vi "SolutionCalculator (SubVI) (2).vi"(4 "Iterative?":bool, 5 "Max Iteration Count":dbl=2.0, 6 "Base Run (matrix)":T1, 7 "Response Coefficients":cdb[][](array[numeric])) -> (0 "Max Residual":dbl, 1 "Correction Phase (radians)":T2, 2 "RMS Residual":dbl format="%0.2f", 3 "Correction Mag":T2)   [LabVIEW 2012]
uses:
  <vilib>/Analysis/Matrix/Datatypes/ComplexMatrix.ctl
  <vilib>/Analysis/Matrix/Datatypes/RealMatrix.ctl
  <vilib>/Analysis/baseanly.llb/Complex A x B.vi
  <vilib>/Analysis/baseanly.llb/Complex Inverse Matrix.vi
  <vilib>/Analysis/Matrix/Numeric/Add/Add - CM,CM.vi
  <vilib>/Analysis/Matrix/Numeric/Conversions/Matrix To Array - CM.vi
  <vilib>/Analysis/5stat.llb/RMS (DBL).vi
  <vilib>/Analysis/Matrix/Numeric/Complex/Complex To Polar - CM.vi
  <vilib>/Analysis/Matrix/Numeric/Absolute Value/Absolute Value - CM.vi
  <vilib>/Analysis/NI_AALBase.lvlib
  <vilib>/Analysis/Matrix/NI_Matrix.lvlib
  <vilib>/Analysis/NI_AALPro.lvlib
panel:
  out "A x B":T1
  out "Epsilon/R":T2
  out "Epsilon":T1
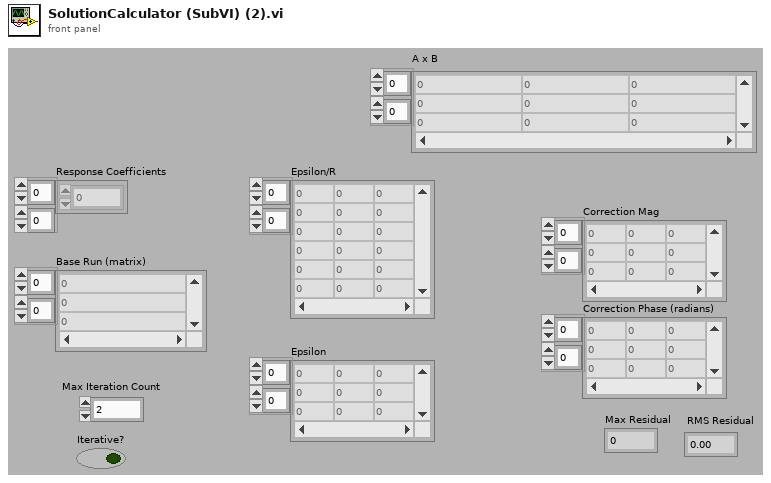
[diagram p1: front panel]
types:
  T1 = typedef "NI_Matrix.lvlib/ComplexMatrix.ctl" = cdb[][]
  T2 = typedef "NI_Matrix.lvlib/RealMatrix.ctl" = dbl[][]
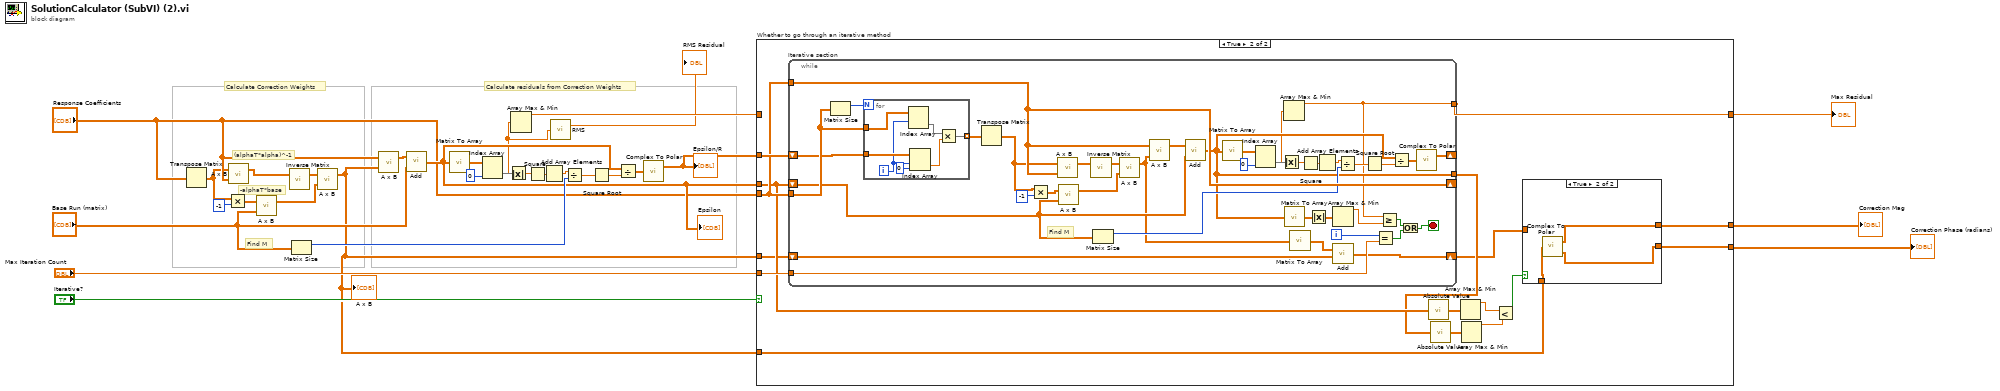
[diagram p0: block diagram]
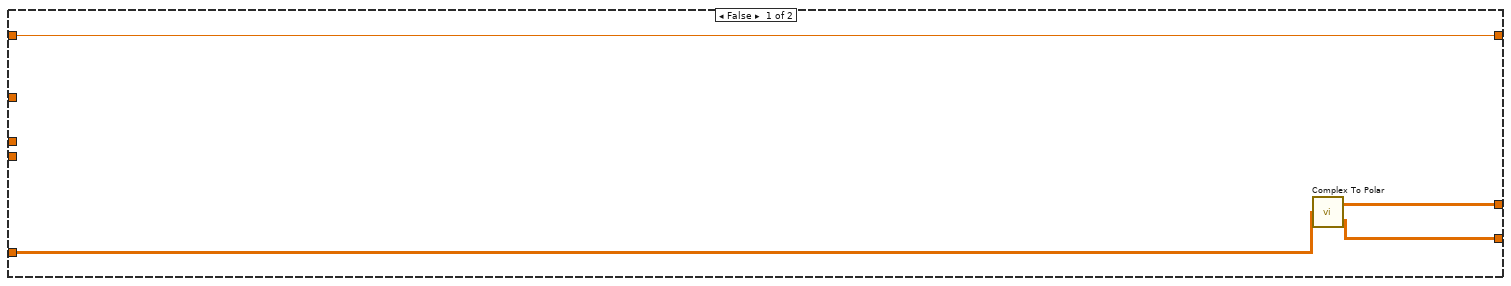
[diagram p2: hidden frame]
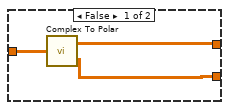
[diagram p3: hidden frame]
diagram:
  # "Calculate residuals from Correction Weights"
  # "Calculate Correction Weights"
  # "-alphaT*base"
  # "(alphaT*alpha)^-1"
  # "Find M"
  n1 = Transpose Matrix(1:"Response Coefficients") -> (0:w6:cdb[][])
  n2 = Multiply ("Multiply.vi")(x=w6, y=-1) -> (x*y=w5:cdb[][])
  n3 = call-poly <vilib>:"A x B.vi"("B"="Response Coefficients", "A"=w6) -> ("A x B"=w4:T1)  [unwired: 1 out]
  n4 = call-poly <vilib>:"A x B.vi"("B"="Base Run (matrix)", "A"=w5) -> ("A x B"=w18:T1)  [unwired: 1 out]
  n5 = call-poly <vilib>:"Inverse Matrix.vi"("Input Matrix"=w4) -> ("Inverse Matrix"=w17:T1)  [unwired: 1 in, 1 out]
  n6 = Matrix Size(0:"Base Run (matrix)") -> (1:w29:i32)  [unwired: 1 out]
  n7 = call-poly <vilib>:"A x B.vi"("B"=w18, "A"=w17) -> ("A x B"=w3:T1)  [unwired: 1 out]
  "A x B" <- w3
  n8 = call-poly <vilib>:"A x B.vi"("B"=w3, "A"="Response Coefficients") -> ("A x B"=w19:T1)  [unwired: 1 out]
  n9 = call-poly <vilib>:"Add.vi"("Complex Matrix B"="Base Run (matrix)", "Complex Matrix A"=w19) -> ("A + B"=w14:T1)
  "Epsilon" <- w14
  n10 = call-poly <vilib>:"Matrix To Array.vi"("Complex Matrix"=w14) -> ("Complex 2D Array"=w20:cdb[][])
  n11 = Index Array(array=w20, index (col)=0 ("disabled index (col)")) -> (element=w27:cdb[])  [unwired: 1 in]
  n12 = Absolute Value(x=w27) -> (abs(x)=w2:dbl[])
  n13 = Array Max & Min(array=w2) -> (max value=w11:dbl)  [unwired: 3 out]
  n14 = Square(x=w2) -> (x^2=w22:dbl[])
  n15 = Add Array Elements(numeric array=w22) -> (sum=w23:dbl)
  n16 = call-poly <vilib>:"RMS.vi"("X"=w2) -> ("rms value"=→"RMS Residual":dbl)  [unwired: 1 out]
  n17 = Divide(x=w23, y=w29) -> (x/y=w24:dbl)
  n18 = Square Root(x=w24) -> (sqrt(x)=w25:dbl)
  n19 = Divide(x=w14, y=w25) -> (x/y=w26:T1)
  n20 = call-poly <vilib>:"Complex To Polar.vi"("Complex Matrix r*e^iQ"=w26) -> ("Modulus r"=w15:T2)  [unwired: 1 out]
  "Epsilon/R" <- w15
  n21 = case "Whether to go through an iterative method" shown="True" "Iterative?" {
    tunnel: "Max Iteration Count" -> [_ w49]
    tunnel: w15 -> [_ w48]
    tunnel: w14 -> [_ w40]
    tunnel: "Response Coefficients" -> [_ w47]
    tunnel: w11 -> [w33 _]
    tunnel: [w33 w46] -> w10
    tunnel: w3 -> [w32 w35]
    tunnel: [w31 w37] -> w9
    tunnel: [w30 w36] -> w8
    tunnel: w3 -> [_ w34]
    frame False {
      n22 = call-poly <vilib>:"Complex To Polar.vi"("Complex Matrix r*e^iQ"=w32) -> ("Modulus r"=w31:T2, "Argument Q"=w30:T2)
    }
    frame True {
      n23 = while "Iterative section" {
        tunnel: w47 -> [w91]
        shift-right: [w65] -> _
        shift-left: w48 -> [w90]
        shift-right: [w66] -> _
        shift-left: w40 -> [w67]
        shift-right: [w80] -> w38
        shift-left: w35 -> [w79]
        tunnel: w49 -> [w81]
        tunnel: w47 -> [w66]
        tunnel: [w61] -> w46
        tunnel: [w63] -> w39
        i -> [w83]
        stop <- w82 stop-if-true
        # "Find M"
        n24 = Matrix Size(0:w91) -> (1:w93:i32)  [unwired: 1 out]
        n25 = for {
          N: w93 -> [_]
          tunnel: w91 -> [w97]
          tunnel: w90 -> [w100]
          tunnel: [w98] -> w92 mode=indexing
          i -> [w94]
          n26 = Index Array(array=w97, index (row)=w94) -> (element=w96:cdb[])  [unwired: 1 in]
          n27 = Index Array(array=w100, index (row)=w94, index (col)=0 ("disabled index (col)")) -> (element=w99:dbl)
          n28 = Multiply(x=w96, y=w99) -> (x*y=w98:cdb[])
        }
        n29 = Transpose Matrix(1:w92) -> (0:w57:cdb[][])
        n30 = Multiply ("Multiply.vi")(x=w57, y=-1) -> (x*y=w59:cdb[][])
        n31 = call-poly <vilib>:"A x B.vi"("B"=w66, "A"=w57) -> ("A x B"=w58:T1)  [unwired: 1 out]
        n32 = call-poly <vilib>:"A x B.vi"("B"=w67, "A"=w59) -> ("A x B"=w77:T1)  [unwired: 1 out]
        n33 = call-poly <vilib>:"Inverse Matrix.vi"("Input Matrix"=w58) -> ("Inverse Matrix"=w78:T1)  [unwired: 1 in, 1 out]
        n34 = Matrix Size(0:w67) -> (1:w64:i32)  [unwired: 1 out]
        n35 = call-poly <vilib>:"A x B.vi"("B"=w77, "A"=w78) -> ("A x B"=w62:T1)  [unwired: 1 out]
        n36 = call-poly <vilib>:"A x B.vi"("B"=w62, "A"=w66) -> ("A x B"=w76:T1)  [unwired: 1 out]
        n37 = call-poly <vilib>:"Add.vi"("Complex Matrix B"=w67, "Complex Matrix A"=w76) -> ("A + B"=w63:T1)
        n38 = call-poly <vilib>:"Matrix To Array.vi"("Complex Matrix"=w63) -> ("Complex 2D Array"=w75:cdb[][])
        n39 = Index Array(array=w75, index (col)=0 ("disabled index (col)")) -> (element=w68:cdb[])  [unwired: 1 in]
        n40 = Absolute Value(x=w68) -> (abs(x)=w56:dbl[])
        n41 = Array Max & Min(array=w56) -> (max value=w61:dbl)  [unwired: 3 out]
        n42 = call-poly <vilib>:"Matrix To Array.vi"("Complex Matrix"=w63) -> ("Complex 2D Array"=w85:cdb[][])
        n43 = call-poly <vilib>:"Matrix To Array.vi"("Complex Matrix"=w62) -> ("Complex 2D Array"=w84:cdb[][])
        n44 = Square(x=w56) -> (x^2=w73:dbl[])
        n45 = Absolute Value(x=w85) -> (abs(x)=w86:dbl[][])
        n46 = Add Array Elements(numeric array=w73) -> (sum=w72:dbl)
        n47 = Array Max & Min(array=w86) -> (max value=w89:dbl)  [unwired: 3 out]
        n48 = call-poly <vilib>:"Add.vi"("Complex Matrix B"=w79, "Complex Matrix A"=w84) -> ("A + B"=w80:T1)
        n49 = Divide(x=w72, y=w64) -> (x/y=w71:dbl)
        n50 = Square Root(x=w71) -> (sqrt(x)=w70:dbl)
        n51 = Equal?(x=w83, y=w81) -> (x = y?=w88:bool)
        n52 = Greater Or Equal?(x=w61, y=w89) -> (x >= y?=w87:bool)
        n53 = Divide(x=w63, y=w70) -> (x/y=w69:T1)
        n54 = Or(x=w87, y=w88) -> (x .or. y?=w82:bool)
        n55 = call-poly <vilib>:"Complex To Polar.vi"("Complex Matrix r*e^iQ"=w69) -> ("Modulus r"=w65:T2)  [unwired: 1 out]
      }
      n56 = call-poly <vilib>:"Absolute Value.vi"("Complex Matrix A"=w40) -> ("|A|"=w42:T2)
      n57 = call-poly <vilib>:"Absolute Value.vi"("Complex Matrix A"=w39) -> ("|A|"=w43:T2)
      n58 = Array Max & Min(array=w42) -> (max value=w44:dbl)  [unwired: 3 out]
      n59 = Array Max & Min(array=w43) -> (max value=w45:dbl)  [unwired: 3 out]
      n60 = Less?(x=w44, y=w45) -> (x < y?=w41:bool)
      n61 = case shown="True" w41 {
        tunnel: w38 -> [w51 _]
        tunnel: [w52 w55] -> w37
        tunnel: [w50 w53] -> w36
        tunnel: w34 -> [_ w54]
        frame False {
          n62 = call-poly <vilib>:"Complex To Polar.vi"("Complex Matrix r*e^iQ"=w51) -> ("Modulus r"=w52:T2, "Argument Q"=w50:T2)
        }
        frame True {
          n63 = call-poly <vilib>:"Complex To Polar.vi"("Complex Matrix r*e^iQ"=w54) -> ("Modulus r"=w55:T2, "Argument Q"=w53:T2)
        }
      }
    }
  }
  "Max Residual" <- w10
  "Correction Mag" <- w9
  "Correction Phase (radians)" <- w8
